vi "Periodic Tasks.vi"(8 "error in":errorcluster) -> ()   [LabVIEW 2018]
doc: "This VI runs in parallel to other tasks. It can contain as many user-defined periodic loops as you need. These can carry out PID or other sorts of timed response."
uses:
  <vilib>/Rock Robotics/WPI/DriverStation/WPI_DriverStationRobotMode2.ctl
  <vilib>/Rock Robotics/WPI/Utilities/WPI_GetSetVariantRefNum.vi
  Robot Global Data.vi
  <vilib>/Rock Robotics/Network Tables/NT Write Numeric Array.vi
  <vilib>/Rock Robotics/Network Tables/NT Write Boolean Array.vi
  <vilib>/Rock Robotics/Network Tables/NT Read Number.vi
  <vilib>/Rock Robotics/Network Tables/NT Write String.vi
  <vilib>/Rock Robotics/Network Tables/NT Write Number.vi
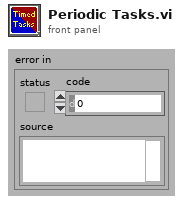
[diagram p1: front panel]
types:
  T1 = typedef "WPI_JoystickDevRef.ctl" = cluster{"Device":T2}
  T2 = typedef "WPI_JoystickDeviceEnum.ctl" = enum16{"USB 0", "USB 1", "USB 2", "USB 3", "USB 4", "USB 5"}
  T3 = typedef "WPI_RobotDriveDevRef.ctl" = cluster{"DevStatus":errorcluster, "Motors[]":T4[], "Square Inputs":bool, "Max Output":dbl}
  T4 = typedef "WPI_MotorControlDeviceRef.ctl" = cluster{"DeviceStatus":errorcluster, "Type":T5, "PWM":cluster{"PWM Channel":T6, "DeadBand":T7}, "CAN":cluster{"Device Number":u8, "SetOutput VI Ref":variant, "GetOutput VI Ref":variant, "Enable VI Ref":variant, "Disable VI Ref":variant, "Data":variant}, "Invert":bool, "DIO PWM":cluster{"PWM \"Enable\" Channel":T6, "DIOChannel":T8, "PWM Rate":dbl}}
  T5 = typedef "WPI_MotorControlType.ctl" = enum16{"PWM", "CAN", "DIO PWM"}
  T6 = typedef "FPGA_DIOPWMChannel.ctl" = enum8{"PWM 0", "PWM 1", "PWM 2", "PWM 3", "PWM 4", "PWM 5", "PWM 6", "PWM 7", "PWM 8", "PWM 9", "PWM MXP 0", "PWM MXP 1", "PWM MXP 2", "PWM MXP 3", "PWM MXP 4", "PWM MXP 5", "PWM MXP 6", "PWM MXP 7", "PWM MXP 8", "PWM MXP 9", "Invalid"}
  T7 = typedef "WPI_PWMDeadband.ctl" = cluster{"Name":string, "maxPositivePwm":i32, "minPositivePwm":i32, "centerPwm":i32, "maxNegativePwm":i32, "minNegativePwm":i32, "angularRange":u16}
  T8 = typedef "FPGA_DIOChannel.ctl" = enum8{"DIO 0", "DIO 1", "DIO 2", "DIO 3", "DIO 4", "DIO 5", "DIO 6", "DIO 7", "DIO 8", "DIO 9", "DIO MXP 0", "DIO MXP 1", "DIO MXP 2", "DIO MXP 3", "DIO MXP 4", "DIO MXP 5", "DIO MXP 6", "DIO MXP 7", "DIO MXP 8", "DIO MXP 9", "DIO MXP 10", "DIO MXP 11", "DIO MXP 12", "DIO MXP 13", "DIO MXP 14", "DIO MXP 15", "SPI Port CS1", "SPI Port CS2", "SPI Port CS3", "SPI Port MISO", "SPI Port MOSI", "Invalid"}
  T9 = typedef "WPI_GyroDevRef.ctl" = cluster{"DevStatus":errorcluster, "Analog Channel":T10, "Gain (VoltsPerDegree/Second)":dbl, "Gyro Type":enum16{"Analog", "XRS450"}, "Handle":i32, "SPI Bus":T11, "Device Found":bool, "Sample Rate":dbl, "Calibrate On Open":bool, "Offset":dbl}
  T10 = typedef "FPGA_AIChannel.ctl" = enum8{"AI 0", "AI 1", "AI 2", "AI 3", "AI MXP 0", "AI MXP 1", "AI MXP 2", "AI MXP 3", "Invalid"}
  T11 = typedef "spi_bus.ctl" = enum16{"SPI On-Board, CS0", "SPI On-Board, CS1", "SPI On-Board, CS2", "SPI On-Board, CS3", "SPI MXP", "Invalid"}
  T12 = cluster{"JoystickDevRef":T1, "JoystickDevRef":T1, "RobotDriveDevRef":T3, "GyroDevRef":T9}
  T13 = typedef "WPI_DriverStationRobotMode2.ctl" = enum16{"Autonomous Disabled", "Autonomous Enabled", "Teleop Disabled", "Teleop Enabled", "Disconnected", "Finish", "Test Disabled", "Test Enabled", "Emergency Stopped"}
  T14 = typedef "WPI_DriverStationPositionInfo.ctl" = enum16{"1", "2", "3"}
  T15 = typedef "WPI_DriverStationAllianceInfo.ctl" = enum16{"Red", "Blue", "Invalid"}
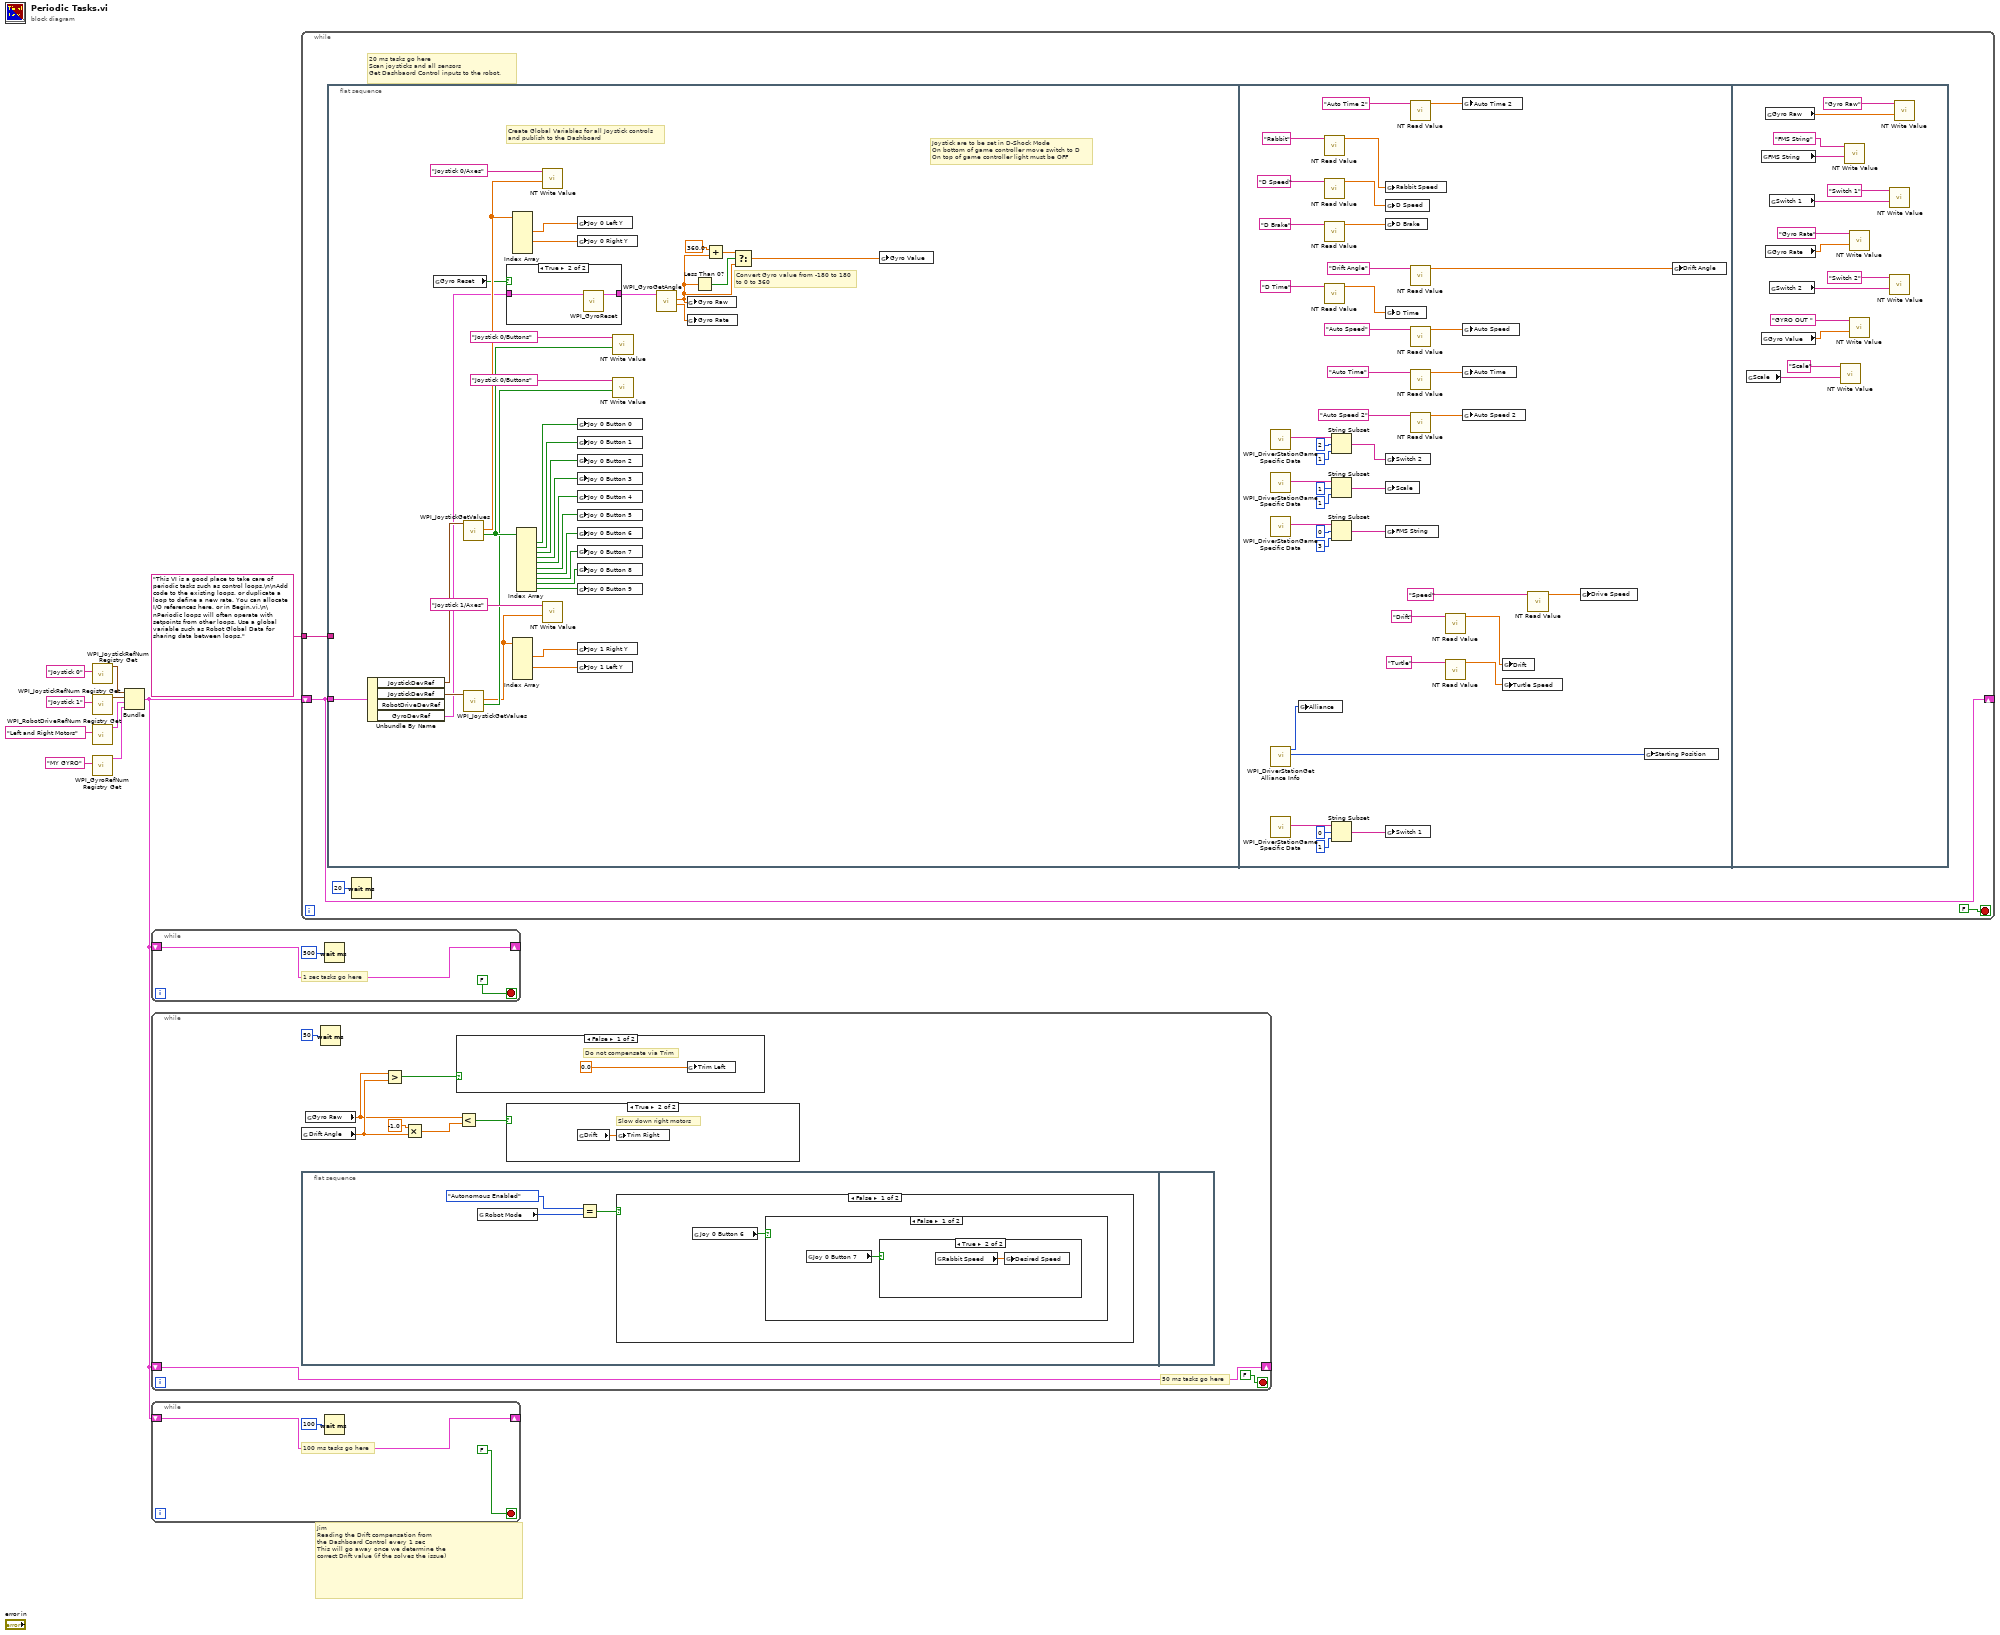
[diagram p0: block diagram]
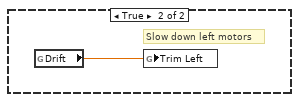
[diagram p2: hidden frame]
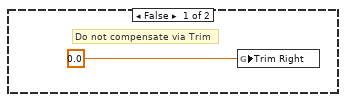
[diagram p3: hidden frame]
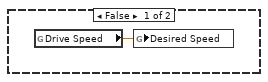
[diagram p4: hidden frame]
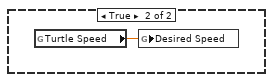
[diagram p5: hidden frame]
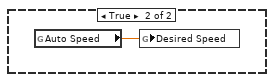
[diagram p6: hidden frame]
diagram:
  # "Jim\nReading the Drift compensation from\nthe Dashboard Control every 1 sec\nThis will go away once we determine the\ncorrect Drift value (if the solves the issue)"
  n1 = call <vilib>:"WPI_JoystickRefNum Registry Get.vi"("refnum name"="Joystick 0") -> ("JoystickDevRef"=w7:T1)  [unwired: 9 in, 1 out]
  n2 = call <vilib>:"WPI_JoystickRefNum Registry Get.vi"("refnum name"="Joystick 1") -> ("JoystickDevRef"=w4:T1)  [unwired: 9 in, 1 out]
  n3 = call <vilib>:"WPI_RobotDriveRefNum Registry Get.vi"("refnum name"="Left and Right Motors") -> ("RobotDriveDevRef"=w6:T3)  [unwired: 1 in, 9 out]
  n4 = call <vilib>:"WPI_GyroRefNum Registry Get.vi"("refnum name"="MY GYRO") -> ("GyroDevRef"=w3:T9)  [unwired: 9 in, 1 out]
  n5 = Bundle("JoystickDevRef"=w7, "JoystickDevRef"=w4, "RobotDriveDevRef"=w6, "GyroDevRef"=w3) -> (w2:T12)  [unwired: 1 out]
  n6 = while {
    shift-right: [w11] -> _
    shift-left: w2 -> [w11]
    stop <- FALSE stop-if-true
    # "1 sec tasks go here"
    n7 = Wait (ms)(milliseconds to wait=u32 500) -> ()  [unwired: 1 out]
  }
  n8 = while {
    shift-right: [w20] -> _
    shift-left: w2 -> [w20]
    stop <- FALSE stop-if-true
    # "50 ms tasks go here"
    n9 = flat-sequence {
      frame #0 {
        n10 = global read "Robot Global Data.vi" "Robot Mode"() -> (w28:T13)
        n11 = Equal?(x=WPI_DriverStationRobotMode2."Autonomous Enabled", y=w28) -> (x = y?=w29:bool)
        n12 = case shown="False" w29 {
          frame False {
            n13 = global read "Robot Global Data.vi" "Joy 0 Button 6"() -> (w30:bool)
            n14 = case shown="False" w30 {
              frame False {
                n15 = global read "Robot Global Data.vi" "Joy 0 Button 7"() -> (w31:bool)
                n16 = case shown="True" w31 {
                  frame False {
                    n17 = global read "Robot Global Data.vi" "Drive Speed"() -> (w32:dbl)
                    n18 = global write "Robot Global Data.vi" "Desired Speed"(w32) -> ()
                  }
                  frame True {
                    n19 = global read "Robot Global Data.vi" "Rabbit Speed"() -> (w33:dbl)
                    n20 = global write "Robot Global Data.vi" "Desired Speed"(w33) -> ()
                  }
                }
              }
              frame True {
                n21 = global read "Robot Global Data.vi" "Turtle Speed"() -> (w34:dbl)
                n22 = global write "Robot Global Data.vi" "Desired Speed"(w34) -> ()
              }
            }
          }
          frame True {
            n23 = global read "Robot Global Data.vi" "Auto Speed"() -> (w35:dbl)
            n24 = global write "Robot Global Data.vi" "Desired Speed"(w35) -> ()
          }
        }
      }
      frame #1 {
      }
    }
    n25 = global read "Robot Global Data.vi" "Drift Angle"() -> (w19:dbl)
    n26 = global read "Robot Global Data.vi" "Gyro Raw"() -> (w17:dbl)
    n27 = Wait (ms)(milliseconds to wait=u32 50) -> ()  [unwired: 1 out]
    n28 = Greater?(x=w17, y=w19) -> (0:w14:bool)
    n29 = Multiply(x=-1.0, y=w19) -> (x*y=w18:dbl)
    n30 = case shown="False" w14 {
      frame False {
        # "Do not compensate via Trim"
        n31 = global write "Robot Global Data.vi" "Trim Left"(0.0 ("Trim Right")) -> ()
      }
      frame True {
        # "Slow down left motors"
        n32 = global read "Robot Global Data.vi" "Drift"() -> (w24:dbl)
        n33 = global write "Robot Global Data.vi" "Trim Left"(w24) -> ()
      }
    }
    n34 = Less?(x=w17, y=w18) -> (x < y?=w15:bool)
    n35 = case shown="True" w15 {
      frame False {
        # "Do not compensate via Trim"
        n36 = global write "Robot Global Data.vi" "Trim Right"(0.0 ("Trim Right")) -> ()
      }
      frame True {
        # "Slow down right motors"
        n37 = global read "Robot Global Data.vi" "Drift"() -> (w26:dbl)
        n38 = global write "Robot Global Data.vi" "Trim Right"(w26) -> ()
      }
    }
  }
  n39 = while {
    shift-right: [w36] -> _
    shift-left: w2 -> [w36]
    stop <- FALSE stop-if-true
    # "100 ms tasks go here"
    n40 = Wait (ms)(milliseconds to wait=u32 100) -> ()  [unwired: 1 out]
  }
  n41 = while {
    shift-right: [w40] -> _
    shift-left: w2 -> [w40]
    tunnel: "This VI is a good place to take care of periodic tasks such as control loops.\n\nAdd code to the existing loops, or duplicate a loop to define a new rate. You can allocate I/O references here, or in Begin.vi.\n\nPeriodic loops will often operate with setpoints from other loops. Use a global variable such as Robot Global Data for sharing data between loops." -> [w39]
    stop <- FALSE stop-if-true
    # "20 ms tasks go here\nScan joysticks and all sensors\nGet Dashbaord Control inputs to the robot."
    n42 = flat-sequence {
      tunnel: w40 -> [w70]
      tunnel: w39 -> [_]
      frame #0 {
        # "Create Global Variables for all Joystick controls\nand publish to the Dashboard"
        # "Convert Gyro value from -180 to 180\nto 0 to 360"
        # "Joystick are to be set in D-Shock Mode\nOn bottom of game controller move switch to D\nOn top of game controller light must be OFF"
        n43 = Unbundle By Name(w70) -> ("JoystickDevRef"=w69:T1, "JoystickDevRef"=w54:T1, "GyroDevRef"=w47:T9)  [unwired: 1 out]
        n44 = global read "Robot Global Data.vi" "Gyro Reset"() -> (w46:bool)
        n45 = call <vilib>:"WPI_JoystickGetValues.vi"("JoystickDevRef"=w69) -> ("Buttons"=w63:bool[], "Axes"=w66:dbl[])  [unwired: 6 in, 3 out]
        n46 = call <vilib>:"WPI_JoystickGetValues.vi"("JoystickDevRef"=w54) -> ("Buttons"=w49:bool[], "Axes"=w43:dbl[])  [unwired: 6 in, 3 out]
        n47 = case shown="True" w46 {
          tunnel: [w77 w79] -> w48
          tunnel: w47 -> [w77 w78]
          frame False {
          }
          frame True {
            n48 = call <vilib>:"WPI_GyroReset.vi"("GyroDevRef"=w78) -> ("GyroDevRef"=w79:T9)  [unwired: 9 in, 1 out]
          }
        }
        n49 = Index Array(array=w66) -> (element #2=w65:dbl, element #4=w64:dbl)  [unwired: 6 in, 4 out]
        n50 = Index Array(array=w43) -> (element #2=w51:dbl, element #4=w52:dbl)  [unwired: 6 in, 4 out]
        n51 = Index Array(array=w63) -> (element #1=w62:bool, element #2=w61:bool, element #3=w60:bool, element #4=w59:bool, element #5=w58:bool, element #6=w57:bool, element #7=w56:bool, element #8=w55:bool, element #9=w45:bool, element #10=w44:bool)  [unwired: 10 in]
        n52 = call-poly <vilib>:"NT Write Value.vi"("Numeric Array"=w66, "Name"="Joystick 0/Axes") -> ()  [unwired: 9 in, 1 out]
        n53 = call-poly <vilib>:"NT Write Value.vi"("Numeric Array"=w43, "Name"="Joystick 1/Axes") -> ()  [unwired: 9 in, 1 out]
        n54 = global write "Robot Global Data.vi" "Joy 0 Left Y"(w65) -> ()
        n55 = global write "Robot Global Data.vi" "Joy 0 Right Y"(w64) -> ()
        n56 = global write "Robot Global Data.vi" "Joy 0 Button 0"(w62) -> ()
        n57 = global write "Robot Global Data.vi" "Joy 0 Button 1"(w61) -> ()
        n58 = global write "Robot Global Data.vi" "Joy 0 Button 2"(w60) -> ()
        n59 = global write "Robot Global Data.vi" "Joy 0 Button 3"(w59) -> ()
        n60 = global write "Robot Global Data.vi" "Joy 0 Button 4"(w58) -> ()
        n61 = global write "Robot Global Data.vi" "Joy 0 Button 5"(w57) -> ()
        n62 = global write "Robot Global Data.vi" "Joy 0 Button 6"(w56) -> ()
        n63 = global write "Robot Global Data.vi" "Joy 0 Button 7"(w55) -> ()
        n64 = global write "Robot Global Data.vi" "Joy 0 Button 8"(w45) -> ()
        n65 = global write "Robot Global Data.vi" "Joy 0 Button 9"(w44) -> ()
        n66 = global write "Robot Global Data.vi" "Joy 1 Right Y"(w51) -> ()
        n67 = global write "Robot Global Data.vi" "Joy 1 Left Y"(w52) -> ()
        n68 = call-poly <vilib>:"NT Write Value.vi"("Boolean Array"=w63, "Name"="Joystick 0/Buttons") -> ()  [unwired: 9 in, 1 out]
        n69 = call-poly <vilib>:"NT Write Value.vi"("Boolean Array"=w49, "Name"="Joystick 0/Buttons") -> ()  [unwired: 9 in, 1 out]
        n70 = call <vilib>:"WPI_GyroGetAngle.vi"("GyroDevRef"=w48) -> ("Angular Rate"=w72:dbl, "Angle"=w71:dbl)  [unwired: 6 in, 3 out]
        n71 = global write "Robot Global Data.vi" "Gyro Raw"(w71) -> ()
        n72 = global write "Robot Global Data.vi" "Gyro Rate"(w72) -> ()
        n73 = Less Than 0?(x=w71) -> (x < 0?=w75:bool)
        n74 = Add(x=360.0 ("y"), y=w71) -> (x+y=w74:dbl)
        n75 = Select(t=w74, s=w75, f=w71) -> (s? t:f=w76:dbl)
        n76 = global write "Robot Global Data.vi" "Gyro Value"(w76) -> ()
      }
      frame #1 {
        n77 = call <vilib>:"WPI_DriverStationGame Specific Data.vi"() -> ("Game Specific Data"=w109:string)  [unwired: 11 in]
        n78 = call <vilib>:"WPI_DriverStationGame Specific Data.vi"() -> ("Game Specific Data"=w108:string)  [unwired: 11 in]
        n79 = call <vilib>:"WPI_DriverStationGame Specific Data.vi"() -> ("Game Specific Data"=w116:string)  [unwired: 11 in]
        n80 = call <vilib>:"WPI_DriverStationGet Alliance Info.vi"() -> ("Position"=w113:T14, "Alliance"=w114:T15)  [unwired: 10 out]
        n81 = call <vilib>:"WPI_DriverStationGame Specific Data.vi"() -> ("Game Specific Data"=w107:string)  [unwired: 11 in]
        n82 = global write "Robot Global Data.vi" "Alliance"(w114) -> ()
        n83 = call-poly <vilib>:"NT Read Value.vi"("Name"="Rabbit") -> ("Numeric"=w118:dbl)  [unwired: 9 in, 1 out]
        n84 = call-poly <vilib>:"NT Read Value.vi"("Name"="D Speed") -> ("Numeric"=w84:dbl)  [unwired: 9 in, 1 out]
        n85 = call-poly <vilib>:"NT Read Value.vi"("Name"="D Brake") -> ("Numeric"=w80:dbl)  [unwired: 9 in, 1 out]
        n86 = call-poly <vilib>:"NT Read Value.vi"("Name"="D Time") -> ("Numeric"=w83:dbl)  [unwired: 9 in, 1 out]
        n87 = String Subset(string=w109, offset (0)=2, length (rest)=1 ("length (rest)")) -> (substring=w112:string)
        n88 = String Subset(string=w108, offset (0)=1, length (rest)=1 ("length (rest)")) -> (substring=w111:string)
        n89 = String Subset(string=w116, offset (0)=0, length (rest)=3 ("length (rest)")) -> (substring=w115:string)
        n90 = String Subset(string=w107, offset (0)=0, length (rest)=1 ("length (rest)")) -> (substring=w110:string)
        n91 = global write "Robot Global Data.vi" "Rabbit Speed"(w118) -> ()
        n92 = global write "Robot Global Data.vi" "D Speed"(w84) -> ()
        n93 = global write "Robot Global Data.vi" "D Brake"(w80) -> ()
        n94 = global write "Robot Global Data.vi" "D Time"(w83) -> ()
        n95 = global write "Robot Global Data.vi" "Switch 2"(w112) -> ()
        n96 = global write "Robot Global Data.vi" "Scale"(w111) -> ()
        n97 = global write "Robot Global Data.vi" "FMS String"(w115) -> ()
        n98 = global write "Robot Global Data.vi" "Switch 1"(w110) -> ()
        n99 = call-poly <vilib>:"NT Read Value.vi"("Name"="Auto Time 2") -> ("Numeric"=w119:dbl)  [unwired: 9 in, 1 out]
        n100 = call-poly <vilib>:"NT Read Value.vi"("Name"="Drift Angle") -> ("Numeric"=w117:dbl)  [unwired: 9 in, 1 out]
        n101 = call-poly <vilib>:"NT Read Value.vi"("Name"="Auto Speed") -> ("Numeric"=w105:dbl)  [unwired: 9 in, 1 out]
        n102 = call-poly <vilib>:"NT Read Value.vi"("Name"="Auto Time") -> ("Numeric"=w106:dbl)  [unwired: 9 in, 1 out]
        n103 = call-poly <vilib>:"NT Read Value.vi"("Name"="Auto Speed 2") -> ("Numeric"=w120:dbl)  [unwired: 9 in, 1 out]
        n104 = call-poly <vilib>:"NT Read Value.vi"("Name"="Drift") -> ("Numeric"=w104:dbl)  [unwired: 9 in, 1 out]
        n105 = call-poly <vilib>:"NT Read Value.vi"("Name"="Turtle") -> ("Numeric"=w121:dbl)  [unwired: 9 in, 1 out]
        n106 = global write "Robot Global Data.vi" "Auto Time 2"(w119) -> ()
        n107 = global write "Robot Global Data.vi" "Auto Speed"(w105) -> ()
        n108 = global write "Robot Global Data.vi" "Auto Time"(w106) -> ()
        n109 = global write "Robot Global Data.vi" "Auto Speed 2"(w120) -> ()
        n110 = global write "Robot Global Data.vi" "Drift"(w104) -> ()
        n111 = global write "Robot Global Data.vi" "Turtle Speed"(w121) -> ()
        n112 = call-poly <vilib>:"NT Read Value.vi"("Name"="Speed") -> ("Numeric"=w87:dbl)  [unwired: 9 in, 1 out]
        n113 = global write "Robot Global Data.vi" "Drive Speed"(w87) -> ()
        n114 = global write "Robot Global Data.vi" "Starting Position"(w113) -> ()
        n115 = global write "Robot Global Data.vi" "Drift Angle"(w117) -> ()
      }
      frame #2 {
        n116 = global read "Robot Global Data.vi" "Scale"() -> (w129:string)
        n117 = global read "Robot Global Data.vi" "FMS String"() -> (w135:string)
        n118 = global read "Robot Global Data.vi" "Gyro Value"() -> (w127:dbl)
        n119 = global read "Robot Global Data.vi" "Gyro Raw"() -> (w126:dbl)
        n120 = global read "Robot Global Data.vi" "Gyro Rate"() -> (w123:dbl)
        n121 = global read "Robot Global Data.vi" "Switch 1"() -> (w133:string)
        n122 = global read "Robot Global Data.vi" "Switch 2"() -> (w132:string)
        n123 = call-poly <vilib>:"NT Write Value.vi"("String"=w129, "Name"="Scale") -> ()  [unwired: 9 in, 1 out]
        n124 = call-poly <vilib>:"NT Write Value.vi"("String"=w135, "Name"="FMS String") -> ()  [unwired: 9 in, 1 out]
        n125 = call-poly <vilib>:"NT Write Value.vi"("Numeric"=w123, "Name"="Gyro Rate") -> ()  [unwired: 9 in, 1 out]
        n126 = call-poly <vilib>:"NT Write Value.vi"("Numeric"=w127, "Name"="GYRO OUT ") -> ()  [unwired: 9 in, 1 out]
        n127 = call-poly <vilib>:"NT Write Value.vi"("String"=w133, "Name"="Switch 1") -> ()  [unwired: 9 in, 1 out]
        n128 = call-poly <vilib>:"NT Write Value.vi"("String"=w132, "Name"="Switch 2") -> ()  [unwired: 9 in, 1 out]
        n129 = call-poly <vilib>:"NT Write Value.vi"("Numeric"=w126, "Name"="Gyro Raw") -> ()  [unwired: 9 in, 1 out]
      }
    }
    n130 = Wait (ms)(milliseconds to wait=u32 20) -> ()  [unwired: 1 out]
  }
